vi "stepper driver -- BLM.vi"(6 "Instrument Address":refnum<visa-resource-name>="ASRL3::INSTR", 7 "stepper driver action":T3=enum."stop", 10 "speed IN":dbl=0.23, 11 "number":dbl=2000.0 format="%#_13g") -> (1 "stepper motor state OUT":T2, 2 "speed":dbl, 3 "number out":dbl)   [LabVIEW 2018]
uses:
  stepper driver action.ctl
  stepper motor state.ctl
  internal stepper driver state -- BLM.ctl
  Q - not nan -- real.vi
panel:
  out "internal stepper driver state BLM OUT":T1={"initialized?"=TRUE, "VISA address"="GPIB0::25::INSTR", "stepper motor state"=enum."moving", "Motor Address"="0", "speed"=0.0, "steps/rot"=8000.0, "vert increment"=0.0042, "target position"=2000.0, "mode"=enum."absolute", "current position"=0.0}
  in  "internal stepper driver state BLM":T1={"initialized?"=TRUE, "VISA address"="GPIB0::25::INSTR", "stepper motor state"=enum."moving", "Motor Address"="0", "speed"=0.0, "steps/rot"=8000.0, "vert increment"=0.0042, "target position"=0.0, "mode"=enum."absolute", "current position"=0.0}
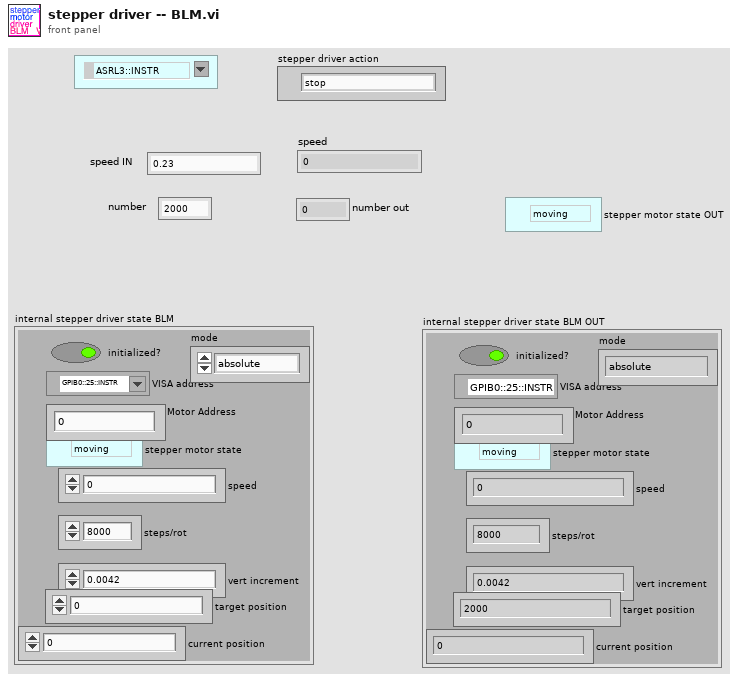
[diagram p1: front panel]
types:
  T1 = typedef "internal stepper driver state -- BLM.ctl" = cluster{"initialized?":bool, "VISA address":refnum<visa-resource-name>, "stepper motor state":T2, "Motor Address":string, "speed":dbl, "steps/rot":dbl, "vert increment":dbl, "target position":dbl, "mode":enum16{"absolute", "relative"}, "current position":dbl}
  T2 = typedef "stepper motor state.ctl" = enum16{"moving", "stopped"}
  T3 = typedef "stepper driver action.ctl" = enum16{"go", "void", "stop", "check", "init", "sync", "set", "set speed", "--check status", "--check value"}
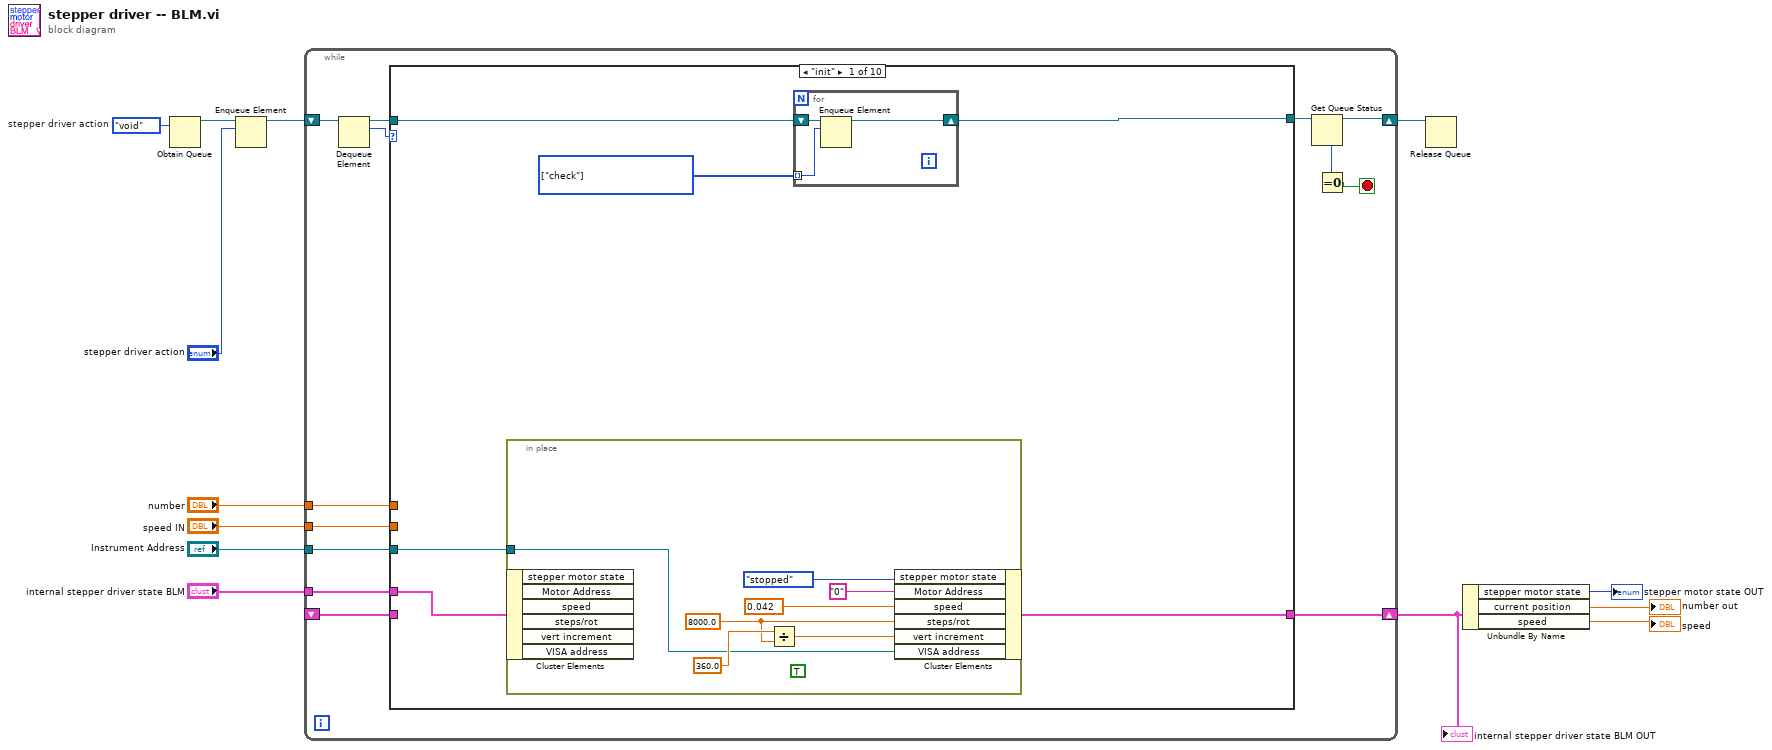
[diagram p0: block diagram]
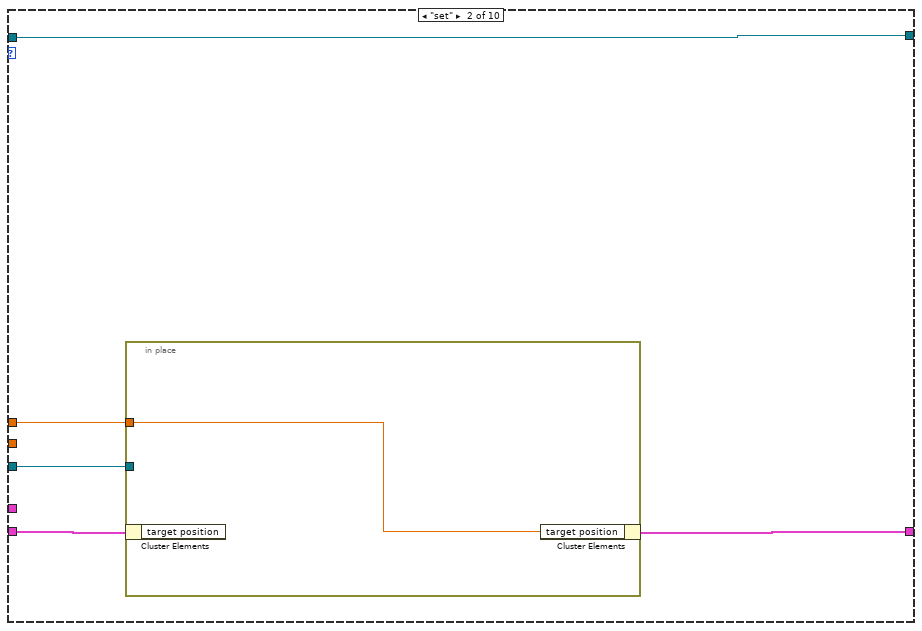
[diagram p2: hidden frame]
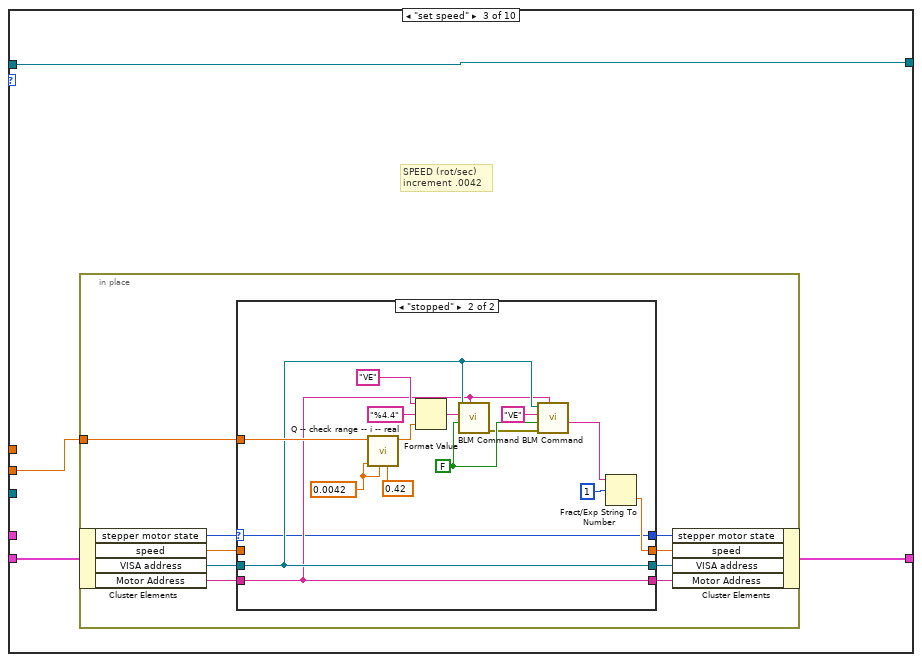
[diagram p3: hidden frame]
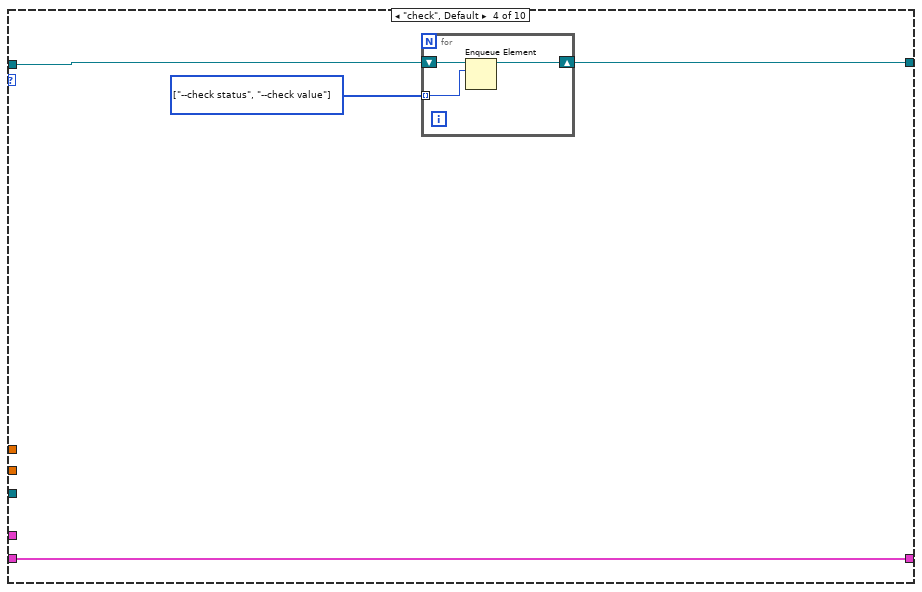
[diagram p5: hidden frame]
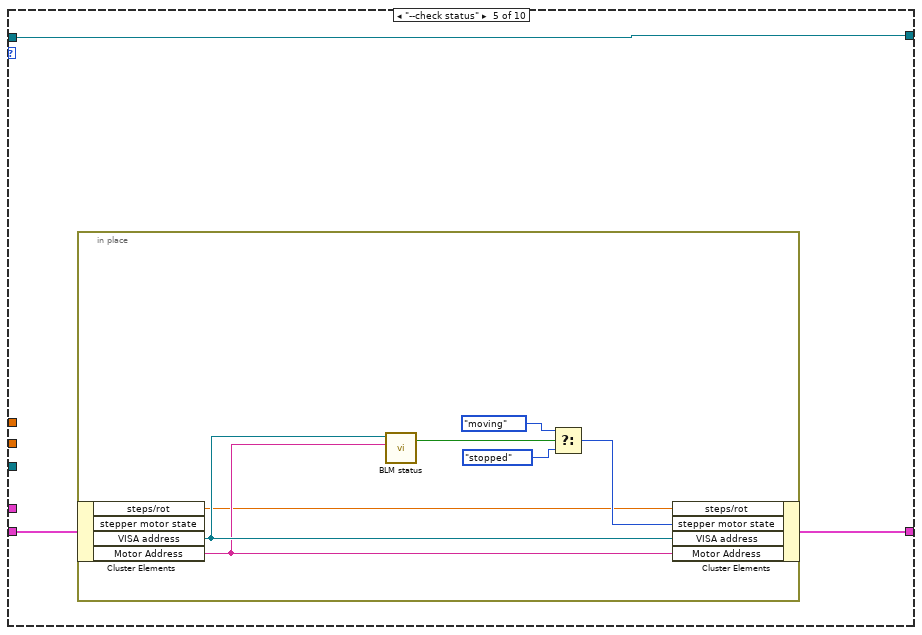
[diagram p6: hidden frame]
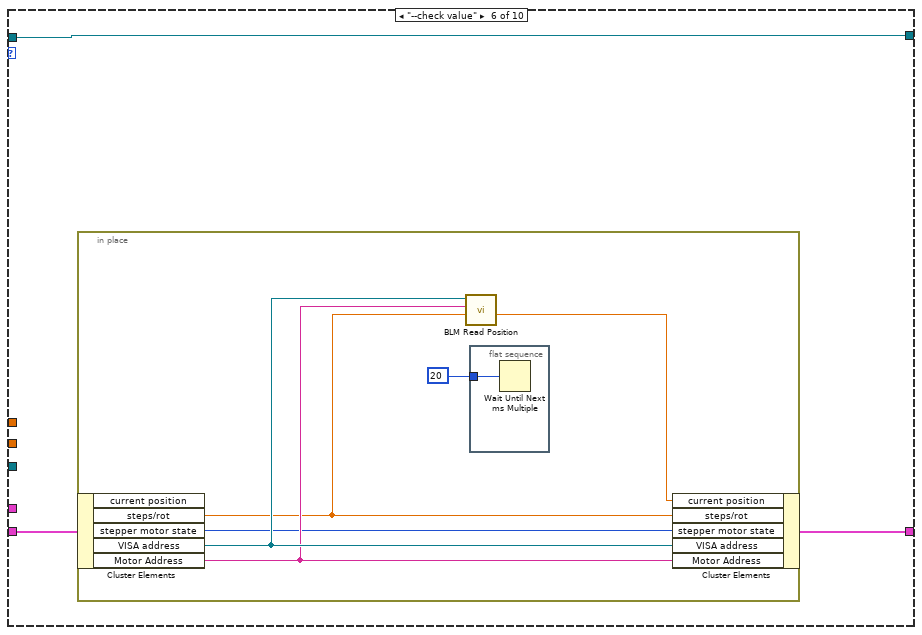
[diagram p7: hidden frame]
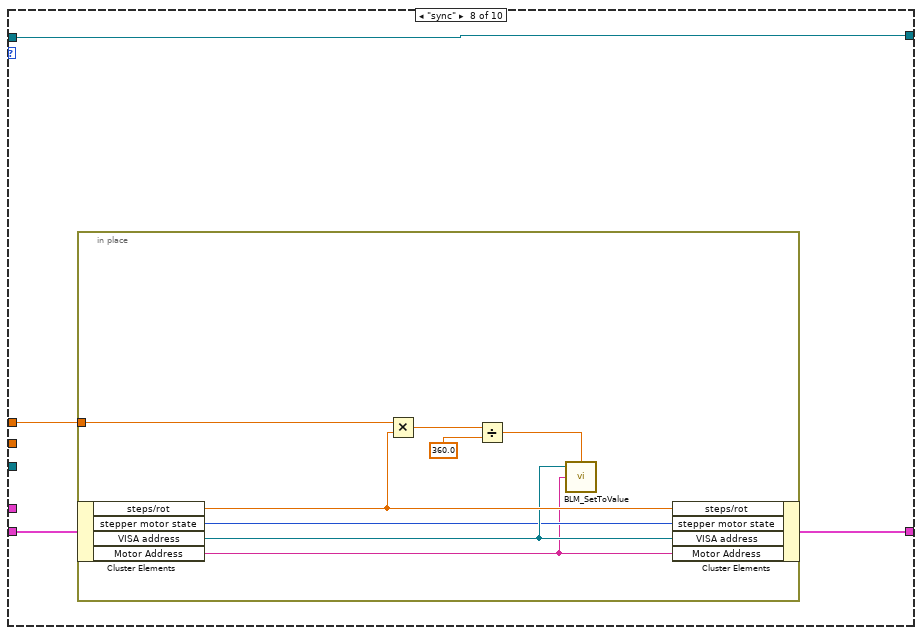
[diagram p9: hidden frame]
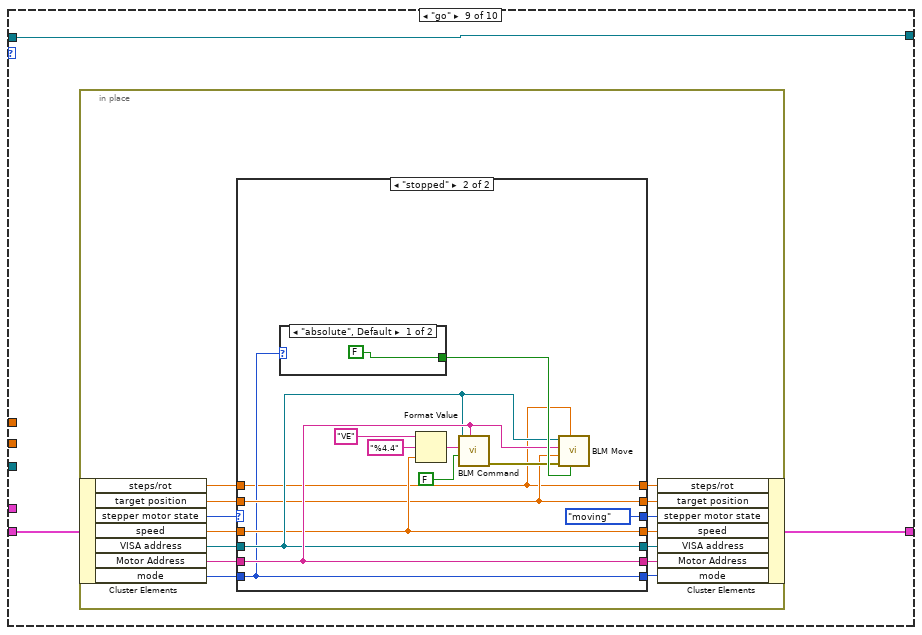
[diagram p10: hidden frame]
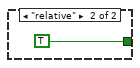
[diagram p12: hidden frame]
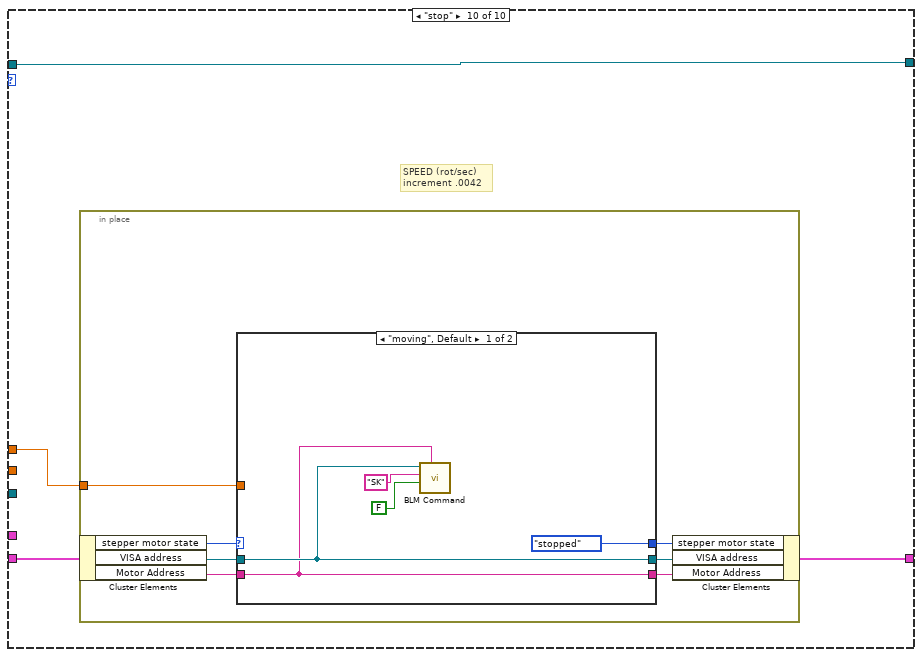
[diagram p13: hidden frame]
diagram:
  w5 = stepper_driver_action."void"  # stepper driver action
  n1 = Obtain Queue(element data type=w5) -> (queue out=w4:refnum<queue>)  [unwired: 4 in, 2 out]
  n2 = Enqueue Element(queue=w4, element="stepper driver action") -> (queue out=w3:refnum<queue>)  [unwired: 2 in, 2 out]
  n3 = while {
    shift-right: [w26] -> w11
    shift-left: _ -> [w25]
    shift-right: [w18] -> w1
    shift-left: w3 -> [w17]
    tunnel: "internal stepper driver state BLM" -> [w24]
    tunnel: "number" -> [w23]
    tunnel: "Instrument Address" -> [w22]
    tunnel: "speed IN" -> [w21]
    stop <- w14 stop-if-true
    n4 = Dequeue Element(queue=w17) -> (queue out=w20:refnum<queue>, element=w16:T3)  [unwired: 2 in, 2 out]
    n5 = case shown="\"init\"" w16 {
      tunnel: [w31 w47 w50 w82 w90 w100 w109 w112 w123 w163] -> w26
      tunnel: w25 -> [_ w43 w51 w82 w91 w101 w109 w113 w124 w164]
      tunnel: [w27 w45 w52 w83 w89 w99 w110 w114 w125 w165] -> w19
      tunnel: w20 -> [w28 w45 w52 w84 w89 w99 w110 w114 w125 w165]
      tunnel: w24 -> [w32 _ _ _ _ _ _ _ _ _]
      tunnel: w23 -> [_ w44 _ _ _ _ _ w111 _ w162]
      tunnel: w22 -> [w30 w46 _ _ _ _ _ _ _ _]
      tunnel: w21 -> [_ _ w49 _ _ _ _ _ _ _]
      frame "init" {
        w29 = T3[] [enum."check"] items=["go", "void", "stop", "check", "init", "sync", "set", "set speed", "--check status", "--check value"] ("action list IN")
        n6 = in-place {
          in-place-border: w30 -> [w36]
          (unwired) TRUE ("something changed")
          w41 = 8000.0 ("Steps/rot")
          n7 = in-place-cluster #1(w32) -> ()  [unwired: 6 out]
          n8 = Divide(x=360.0, y=w41) -> (x/y=w40:dbl)
          n9 = in-place-cluster #1("stepper motor state"=stepper_motor_state."stopped", "Motor Address"="0", "speed"=0.042, "steps/rot"=w41, "vert increment"=w40, "VISA address"=w36) -> (w31:T1)
        }
        n10 = for {
          shift-right: [w34] -> w27
          shift-left: w28 -> [w35]
          tunnel: w29 -> [w33] mode=indexing
          n11 = Enqueue Element(queue=w35, element=w33) -> (queue out=w34:refnum<queue>)  [unwired: 2 in, 2 out]
        }
      }
      frame "set" {
        n12 = in-place {
          in-place-border: w46 -> [_]
          in-place-border: w44 -> [w48]
          n13 = in-place-cluster #2(w43) -> ()  [unwired: 1 out]
          n14 = in-place-cluster #2("target position"=w48) -> (w47:T1)
        }
      }
      frame "set speed" {
        # "SPEED (rot/sec)\nincrement .0042"
        n15 = in-place {
          in-place-border: w49 -> [w61]
          n16 = in-place-cluster #3(w51) -> ("stepper motor state"=w57:T2, "speed"=w56:dbl, "VISA address"=w59:refnum<visa-resource-name>, "Motor Address"=w58:string)
          n17 = case shown="\"stopped\"" w57 {
            selector: w57 -> [w62 w66]
            tunnel: w61 -> [_ w73]
            tunnel: [w65 w69] -> w60
            tunnel: w59 -> [w64 w68]
            tunnel: w58 -> [w63 w67]
            tunnel: w56 -> [w65 _]
            tunnel: [w64 w68] -> w55
            tunnel: [w63 w67] -> w54
            tunnel: [w62 w66] -> w53
            frame "moving", Default {
            }
            frame "stopped" {
              w81 = FALSE
              w72 = 0.0042 ("lower limit")
              n18 = call "Q -- check range -- i -- real.vi"("upper"=0.42 ("x"), "lower"=w72, "default"=w72, "number"=w73) -> ("number in range"=w70:dbl)  [unwired: 5 in, 2 out]
              n19 = Format Value(string ("")="VE", format string="%4.4", value (0)=w70) -> (output string=w77:string)
              n20 = call "BLM Command.vi"("Motor Address"=w67, "Read Echo?"=w81, "Command"=w77, "Port Address"=w68) -> ("error out"=w80:errorcluster)  [unwired: 2 in, 4 out]
              n21 = call "BLM Command.vi"("Motor Address"=w67, "error in (no error)"=w80, "Read Echo?"=w81, "Command"="VE", "Port Address"=w68) -> ("Response"=w75:string)  [unwired: 1 in, 4 out]
              n22 = Fract/Exp String To Number(string=w75, offset=1) -> (number=w69:dbl)  [unwired: 2 in, 1 out]
            }
          }
          n23 = in-place-cluster #3("stepper motor state"=w53, "speed"=w60, "VISA address"=w55, "Motor Address"=w54) -> (w50:T1)
        }
      }
      frame "check", Default {
        w85 = T3[] [enum."--check status", enum."--check value"] items=["go", "void", "stop", "check", "init", "sync", "set", "set speed", "--check status", "--check value"] ("action list IN")
        n24 = for {
          shift-right: [w87] -> w83
          shift-left: w84 -> [w88]
          tunnel: w85 -> [w86] mode=indexing
          n25 = Enqueue Element(queue=w88, element=w86) -> (queue out=w87:refnum<queue>)  [unwired: 2 in, 2 out]
        }
      }
      frame "--check status" {
        n26 = in-place {
          n27 = in-place-cluster #4(w91) -> ("steps/rot"=w92:dbl, "VISA address"=w98:refnum<visa-resource-name>, "Motor Address"=w97:string)  [unwired: 1 out]
          n28 = call "BLM status.vi"("Motor Address"=w97, "Porty Address"=w98) -> ("Motor is moving"=w96:bool)  [unwired: 2 in, 1 out]
          n29 = Select(t=stepper_motor_state."moving" ("stepper motor state"), s=w96, f=stepper_motor_state."stopped" ("stepper motor state")) -> (s? t:f=w93:T2)
          n30 = in-place-cluster #4("steps/rot"=w92, "stepper motor state"=w93, "VISA address"=w98, "Motor Address"=w97) -> (w90:T1)
        }
      }
      frame "--check value" {
        n31 = in-place {
          n32 = in-place-cluster #5(w101) -> ("steps/rot"=w104:dbl, "stepper motor state"=w103:T2, "VISA address"=w107:refnum<visa-resource-name>, "Motor Address"=w106:string)  [unwired: 1 out]
          n33 = call "BLM Read Position.vi"("Steps/rot"=w104, "Motor Address"=w106, "Port Address"=w107) -> ("Response"=w105:dbl)  [unwired: 1 in, 3 out]
          n34 = flat-sequence {
            tunnel: u32 20 ("millisecond multiple") -> [w108]
            frame #0 {
              n35 = Wait Until Next ms Multiple(millisecond multiple=w108) -> ()  [unwired: 1 out]
            }
          }
          n36 = in-place-cluster #5("current position"=w105, "steps/rot"=w104, "stepper motor state"=w103, "VISA address"=w107, "Motor Address"=w106) -> (w100:T1)
        }
      }
      frame "void" {
      }
      frame "sync" {
        n37 = in-place {
          in-place-border: w111 -> [w119]
          n38 = in-place-cluster #6(w113) -> ("steps/rot"=w118:dbl, "stepper motor state"=w116:T2, "VISA address"=w117:refnum<visa-resource-name>, "Motor Address"=w115:string)
          n39 = Multiply(x=w119, y=w118) -> (x*y=w121:dbl)
          n40 = Divide(x=w121, y=360.0) -> (x/y=w122:dbl)
          n41 = call "BLM_SetToValue.vi"("Position"=w122, "Motor Address"=w115, "Port Address"=w117) -> ()  [unwired: 1 in, 1 out]
          n42 = in-place-cluster #6("steps/rot"=w118, "stepper motor state"=w116, "VISA address"=w117, "Motor Address"=w115) -> (w112:T1)
        }
      }
      frame "go" {
        n43 = in-place {
          n44 = in-place-cluster #7(w124) -> ("steps/rot"=w127:dbl, "target position"=w131:dbl, "stepper motor state"=w136:T2, "speed"=w135:dbl, "VISA address"=w138:refnum<visa-resource-name>, "Motor Address"=w137:string, "mode"=w132:enum16{"absolute", "relative"})
          n45 = case shown="\"stopped\"" w136 {
            selector: w136 -> [w141 _]
            tunnel: [w146 w152] -> w139
            tunnel: w138 -> [w145 w153]
            tunnel: w137 -> [w144 w154]
            tunnel: w135 -> [w146 w152]
            tunnel: [w145 w153] -> w134
            tunnel: [w144 w154] -> w133
            tunnel: w132 -> [w140 w148]
            tunnel: w131 -> [w142 w149]
            tunnel: [w141 stepper_motor_state."moving" ("stepper motor state")] -> w130
            tunnel: [w142 w149] -> w129
            tunnel: [w143 w147] -> w128
            tunnel: w127 -> [w143 w147]
            tunnel: [w140 w148] -> w126
            frame "moving", Default {
            }
            frame "stopped" {
              n46 = case shown="\"absolute\", Default" w148 {
                tunnel: [FALSE TRUE] -> w155
                frame "absolute", Default {
                }
                frame "relative" {
                }
              }
              n47 = Format Value(string ("")="VE", format string="%4.4", value (0)=w152) -> (output string=w156:string)
              n48 = call "BLM Command.vi"("Motor Address"=w154, "Read Echo?"=FALSE, "Command"=w156, "Port Address"=w153) -> ("error out"=w151:errorcluster)  [unwired: 2 in, 4 out]
              n49 = call "BLM Move.vi"("Mode IS:"=w155, "Steps/rot"=w147, "error in (no error)"=w151, "Position / Distance"=w149, "Motor Address"=w154, "Port Address"=w153) -> ()  [unwired: 1 out]
            }
          }
          n50 = in-place-cluster #7("steps/rot"=w128, "target position"=w129, "stepper motor state"=w130, "speed"=w139, "VISA address"=w134, "Motor Address"=w133, "mode"=w126) -> (w123:T1)
        }
      }
      frame "stop" {
        # "SPEED (rot/sec)\nincrement .0042"
        n51 = in-place {
          in-place-border: w162 -> [w172]
          n52 = in-place-cluster #8(w164) -> ("stepper motor state"=w169:T2, "VISA address"=w171:refnum<visa-resource-name>, "Motor Address"=w170:string)
          n53 = case shown="\"moving\", Default" w169 {
            selector: w169 -> [_ w178]
            tunnel: w172 -> [_ _]
            tunnel: w171 -> [w175 w180]
            tunnel: w170 -> [w174 w179]
            tunnel: [w175 w180] -> w168
            tunnel: [w174 w179] -> w167
            tunnel: [stepper_motor_state."stopped" ("stepper motor state") w178] -> w166
            frame "moving", Default {
              n54 = call "BLM Command.vi"("Motor Address"=w174, "Read Echo?"=FALSE, "Command"="SK", "Port Address"=w175) -> ()  [unwired: 2 in, 5 out]
            }
            frame "stopped" {
            }
          }
          n55 = in-place-cluster #8("stepper motor state"=w166, "VISA address"=w168, "Motor Address"=w167) -> (w163:T1)
        }
      }
    }
    n56 = Get Queue Status(queue=w19) -> (queue out=w18:refnum<queue>, # elements in queue=w15:i32)  [unwired: 2 in, 6 out]
    n57 = Equal To 0?(x=w15) -> (x = 0?=w14:bool)
  }
  "internal stepper driver state BLM OUT" <- w11
  n58 = Release Queue(queue=w1) -> ()  [unwired: 2 in, 3 out]
  n59 = Unbundle By Name(w11) -> ("stepper motor state"=→"stepper motor state OUT":T2, "current position"=→"number out":dbl, "speed"=→"speed":dbl)
